vi "Init.vi"(5 "PathControl.lvclass":refnum<class "PathControl.lvclass">, 6 "Environmental classes":refnum<class "Instrument.lvclass">[](array[class]), 7 "XML Handler.lvclass":refnum<class "XML Handler.lvclass">, 8 "error in (no error)":errorcluster, 9 "Instruments to Use":T1(array[cluster]), 10 "Device.lvclass":refnum<class "Device.lvclass">, 11 "RF Powers in":refnum<class "RF Power.lvclass">) -> (0 "error out":errorcluster, 3 "RF Powers out":refnum<class "RF Power.lvclass">)   [LabVIEW 2020, in "RF Power.lvclass"]
doc: "Initializes the measurement.\nThis verifies that the instruments are present and adds them into the class data.\nIs also adds the xml handler into the class data."
uses:
  RF Power.lvclass
  Devices/Device.lvclass
  Instruments/Instrument.lvclass
  XML Handler/XML Handler.lvclass
  Path Control/PathControl.lvclass
  Harmonics/Controls/Init states.ctl
  Instruments/Signal Generator/Signal Generator.lvclass
  Instruments/Power Meter/Power Meter.lvclass
  Measurement.lvclass
  Harmonics/Harmonics.lvclass
panel:
  out "Current State":string
  out "Initializing Harmonic Measurement":u8(slide) scale=0.0..100.0
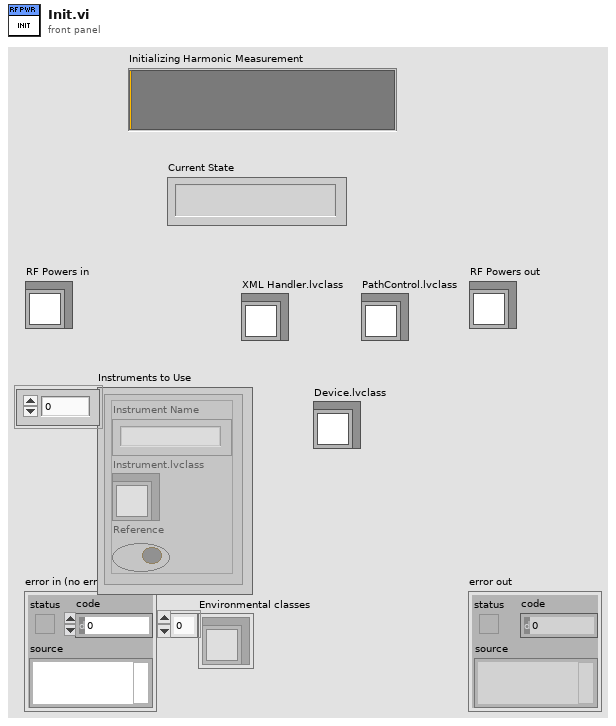
[diagram p1: front panel]
types:
  T1 = cluster{"Instrument Name":string, "Instrument.lvclass":refnum<class "Instrument.lvclass">, "Reference":bool}[]
  T2 = typedef "Harmonics.lvclass/Init states.ctl" = enum16{"Verify instruments", "Init Sweep Parameters", "Init Instruments", "Done"}
  T3 = typedef "RF Power.lvclass/Config info.ctl" = cluster{"Frequency (MHz)":string, "Power (dBm)":string, "Loop order":T4, "SG loss":bool, "PM loss":bool, "SG":i32}
  T4 = typedef "RF Power.lvclass/Loop order.ctl" = enum16{"Device -> Power -> Frequency", "Device -> Frequency -> Power"}
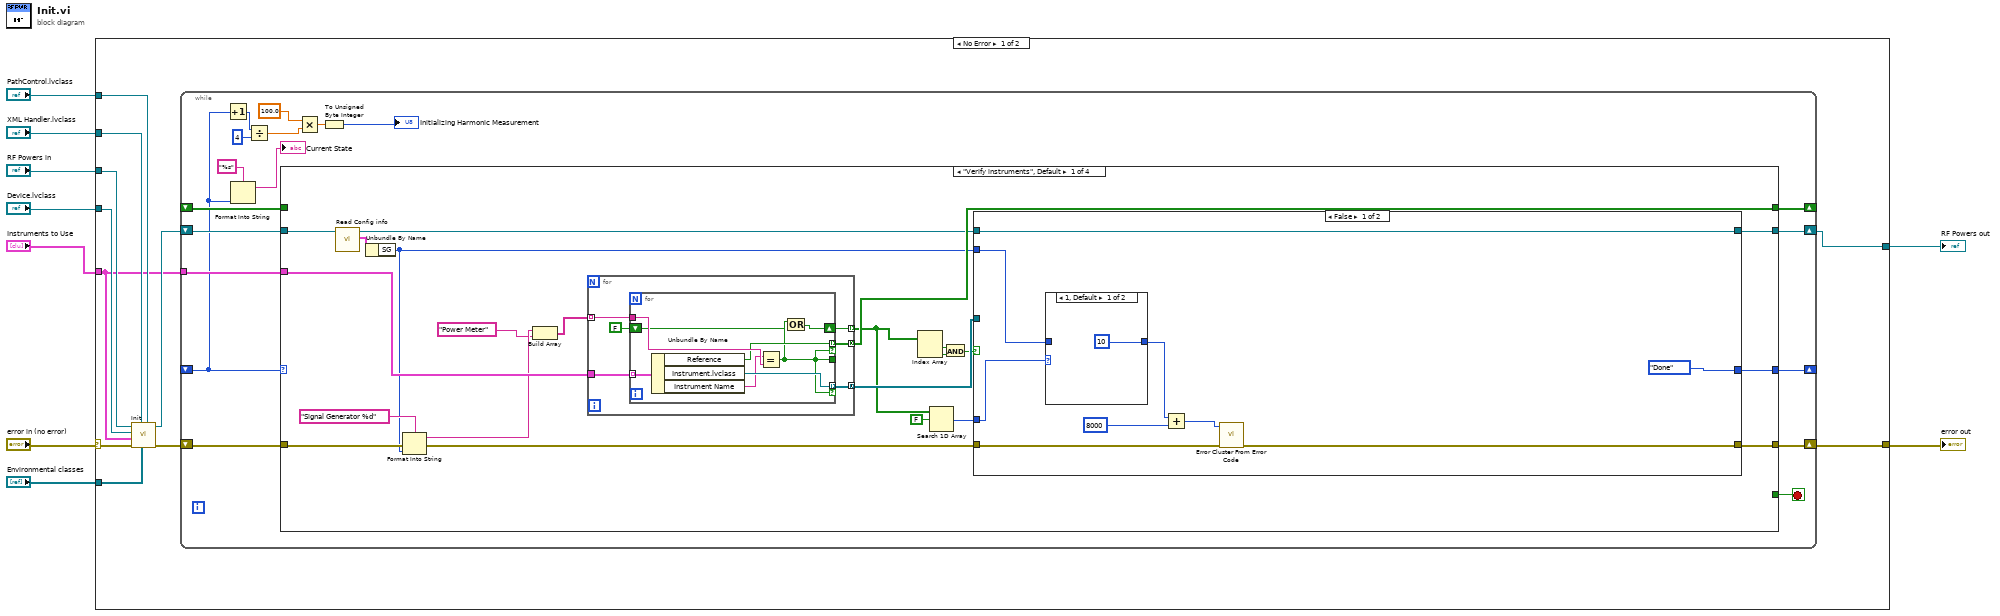
[diagram p0: block diagram]
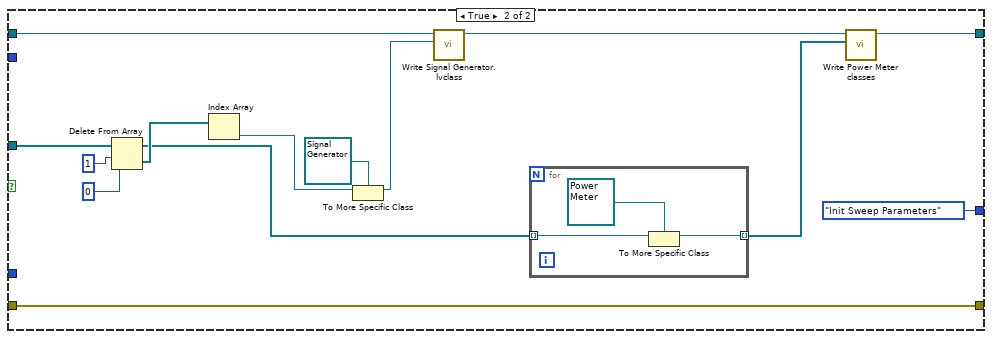
[diagram p3: hidden frame]
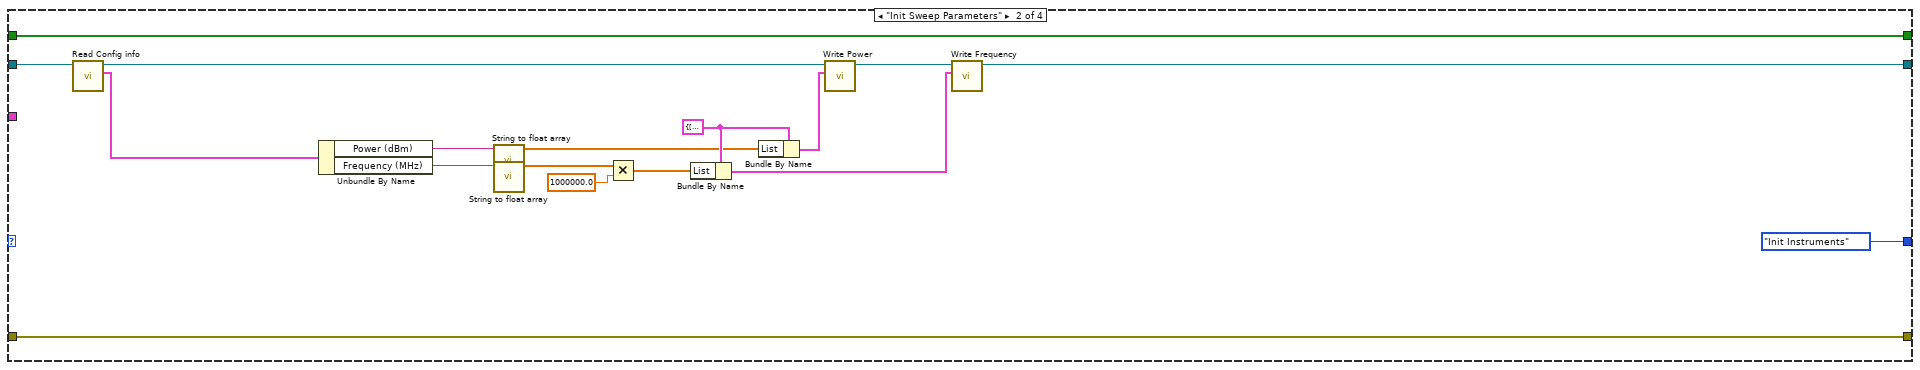
[diagram p4: hidden frame]
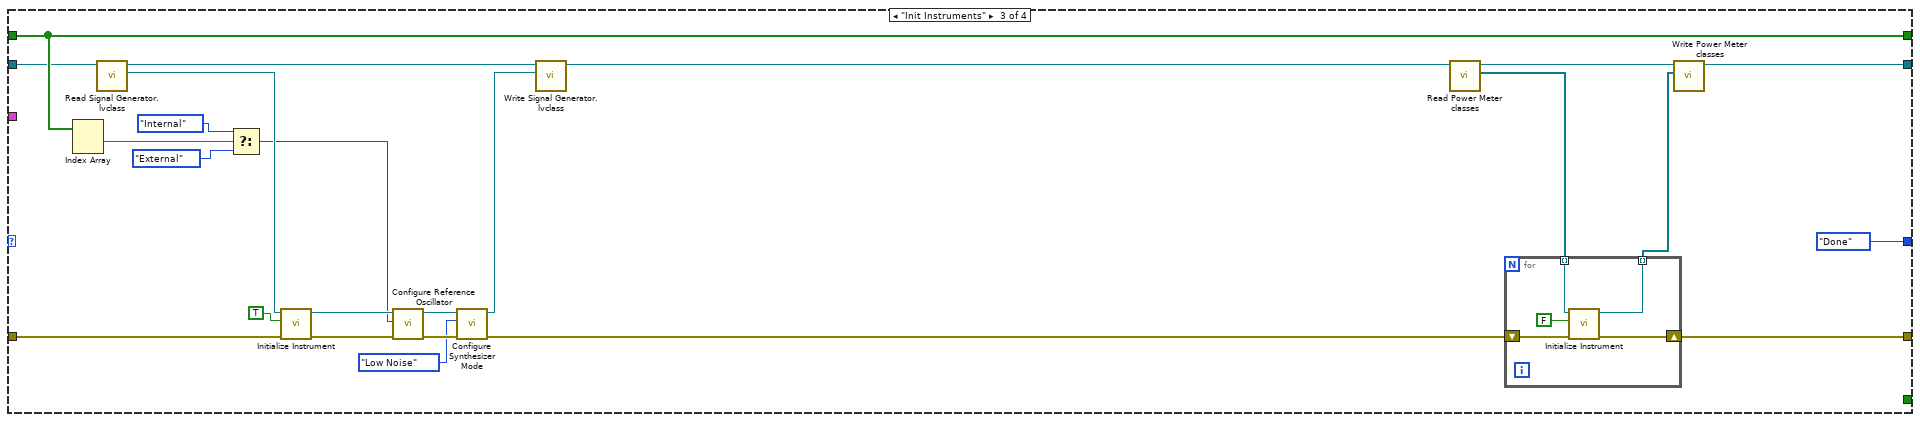
[diagram p5: hidden frame]
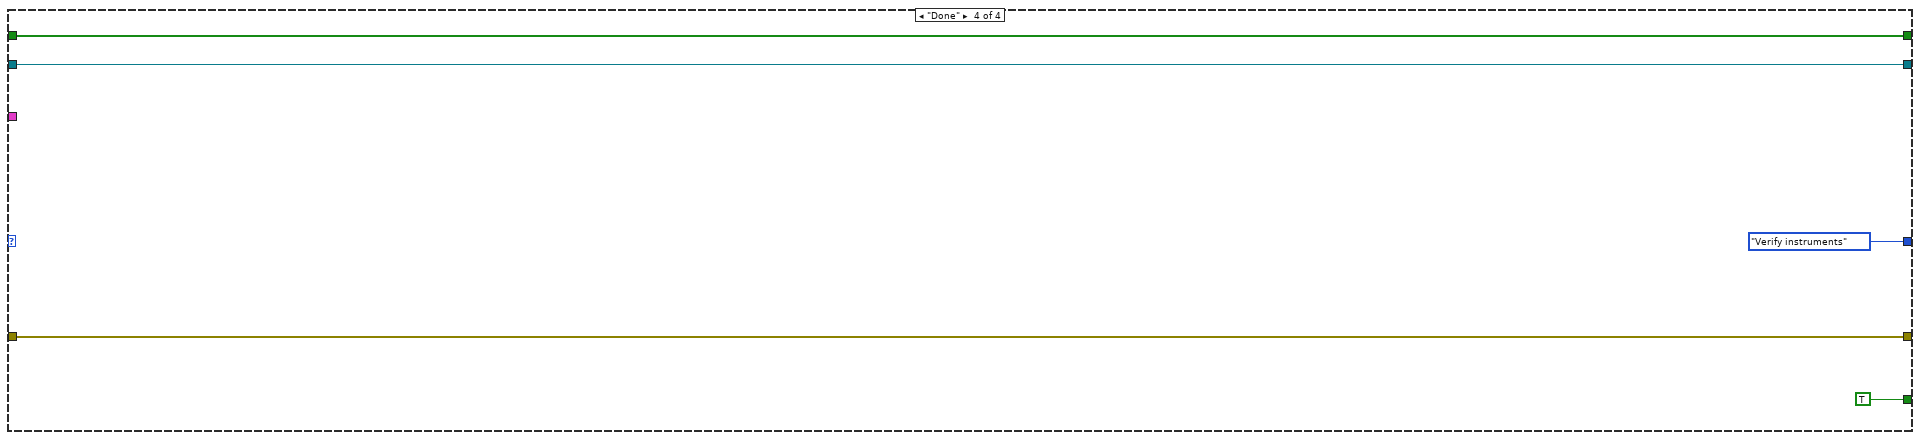
[diagram p6: hidden frame]
diagram:
  n1 = case shown="No Error" "error in (no error)" {
    selector: "error in (no error)" -> [w17 w154]
    tunnel: "PathControl.lvclass" -> [w20 _]
    tunnel: "Environmental classes" -> [w19 _]
    tunnel: "XML Handler.lvclass" -> [w18 _]
    tunnel: "Device.lvclass" -> [w16 _]
    tunnel: "RF Powers in" -> [w15 w155]
    tunnel: [w13 w154] -> w3
    tunnel: "Instruments to Use" -> [w11 _]
    tunnel: [w10 w155] -> w1
    frame No Error {
      n2 = call-parent "Init.vi"("PathControl.lvclass"=w20, "Environmental classes"=w19, "XML Handler.lvclass"=w18, "error in (no error)"=w17, "Instruments to Use"=w11, "Device.lvclass"=w16, "Measurements in"=w15) -> ("error out"=w14:errorcluster, "Measurements out"=w12:refnum<class "RF Power.lvclass">)  [unwired: 3 in]
      n3 = while {
        shift-right: [w34] -> w13
        shift-left: w14 -> [w35]
        tunnel: w11 -> [w38]
        shift-right: [w36] -> w10
        shift-left: w12 -> [w37]
        shift-right: [w32] -> _
        shift-left: _ -> [w27]
        shift-right: [w31] -> _
        shift-left: _ -> [w30]
        stop <- w33 stop-if-true
        n4 = Increment(x=w27) -> (x+1=w26:T2)
        n5 = Format Into String(format string="%s", w27) -> (resulting string=→"Current State":string)  [unwired: 2 in, 1 out]
        n6 = Divide(x=w26, y=4) -> (x/y=w24:dbl)
        n7 = case shown="\"Verify instruments\", Default" w27 {
          tunnel: w38 -> [w57 _ _ _]
          tunnel: w37 -> [w48 w104 w130 w149]
          tunnel: [w60 w106 w124 w149] -> w36
          tunnel: w35 -> [w44 w118 w142 w151]
          tunnel: [w59 w118 w131 w151] -> w34
          tunnel: [w58 Init_states."Init Instruments" Init_states."Done" Init_states."Verify instruments"] -> w32
          tunnel: [_ _ _ TRUE] -> w33
          tunnel: [w52 w116 w140 w153] -> w31
          tunnel: w30 -> [_ w116 w140 w153]
          frame "Verify instruments", Default {
            n8 = call-dynamic "Read Config info.vi"("RF Power in"=w48) -> ("Config info"=w45:T3, "RF Power out"=w47:refnum<class "RF Power.lvclass">)  [unwired: 9 in]
            n9 = Unbundle By Name(w45) -> ("SG"=w39:i32)
            n10 = Format Into String(format string="Signal Generator %d", error in=w44, w39) -> (resulting string=w42:string, error out=w43:errorcluster)  [unwired: 1 in]
            n11 = Build Array(w42, "Power Meter") -> (w40:string[])
            n12 = for {
              tunnel: [w66] -> w56 mode=concatenating
              tunnel: [w61] -> w51 mode=indexing
              tunnel: [w65] -> w52 mode=concatenating
              tunnel: w40 -> [w64] mode=indexing
              tunnel: w57 -> [w63]
              n13 = for {
                tunnel: w63 -> [w71] mode=indexing
                tunnel: w64 -> [w74]
                tunnel: [w73] -> w66 mode=indexing if=w68
                tunnel: [w68] -> _
                tunnel: [w72] -> w65 mode=indexing if=w68
                shift-right: [w69] -> w61
                shift-left: FALSE -> [w67]
                n14 = Unbundle By Name(w71) -> ("Reference"=w72:bool, "Instrument.lvclass"=w73:refnum<class "Instrument.lvclass">, "Instrument Name"=w70:string)
                n15 = Equal?(x=w70, y=w74) -> (x = y?=w68:bool)
                n16 = Or(x=w68, y=w67) -> (x .or. y?=w69:bool)
              }
            }
            n17 = Index Array(array=w51) -> (element #1=w55:bool, element #2=w54:bool)  [unwired: 2 in]
            n18 = Search 1D Array(1D array=w51, element=FALSE) -> (index of element=w49:i32)  [unwired: 1 in]
            n19 = And(x=w55, y=w54) -> (x .and. y?=w53:bool)
            n20 = case shown="False" w53 {
              tunnel: w56 -> [_ w93]
              tunnel: w47 -> [w83 w89]
              tunnel: [w83 w87] -> w60
              tunnel: w43 -> [w82 w96]
              tunnel: [w79 w96] -> w59
              tunnel: [Init_states."Done" Init_states."Init Sweep Parameters"] -> w58
              tunnel: w49 -> [w77 _]
              tunnel: w39 -> [w76 _]
              frame False {
                n21 = case shown="1, Default" w77 {
                  tunnel: w76 -> [_ w85]
                  tunnel: [10 ("y") w85] -> w75
                  frame 1, Default {
                  }
                  frame 0 {
                  }
                }
                n22 = Add(x=w75, y=8000) -> (x+y=w80:i32)
                n23 = call <vilib>:"Error Cluster From Error Code.vi"("error in (no error)"=w82, "error code (0)"=w80) -> ("error out"=w79:errorcluster)  [unwired: 7 in]
              }
              frame True {
                n24 = Delete From Array(array=w93, length=1, index=0) -> (deleted portion=w92:refnum<class "Instrument.lvclass">[], array with subset deleted=w91:refnum<class "Instrument.lvclass">[])
                n25 = Index Array(array=w92) -> (element=w99:refnum<class "Instrument.lvclass">)  [unwired: 1 in]
                n26 = To More Specific Class(target class=refnum<class "Signal Generator.lvclass"> refnum ("Signal Generator.lvclass"), reference=w99) -> (specific class reference=w90:refnum<class "Signal Generator.lvclass">)  [unwired: 1 in, 1 out]
                n27 = call-dynamic "Write Signal Generator.lvclass.vi"("Signal Generator.lvclass"=w90, "RF Power in"=w89) -> ("RF Power out"=w88:refnum<class "RF Power.lvclass">)  [unwired: 9 in]
                n28 = for {
                  tunnel: [w101] -> w86 mode=indexing
                  tunnel: w91 -> [w100] mode=indexing
                  n29 = To More Specific Class(target class=refnum<class "Power Meter.lvclass"> refnum ("Power Meter.lvclass"), reference=w100) -> (specific class reference=w101:refnum<class "Power Meter.lvclass">)  [unwired: 1 in, 1 out]
                }
                n30 = call-dynamic "Write Power Meter classes.vi"("Power Meter classes"=w86, "RF Power in"=w88) -> ("RF Power out"=w87:refnum<class "RF Power.lvclass">)  [unwired: 9 in]
              }
            }
          }
          frame "Init Sweep Parameters" {
            w117 = cluster{"List":dbl[], "Index":i32, "Last":bool} {"List"=[], "Index"=0, "Last"=FALSE} ("Power")
            n31 = call-dynamic "Read Config info.vi"("RF Power in"=w104) -> ("Config info"=w109:T3, "RF Power out"=w103:refnum<class "RF Power.lvclass">)  [unwired: 9 in]
            n32 = Unbundle By Name(w109) -> ("Power (dBm)"=w113:string, "Frequency (MHz)"=w111:string)
            n33 = call "String to float array.vi"("String"=w113) -> ("Array - Numeric"=w112:dbl[])  [unwired: 9 in, 1 out]
            n34 = call "String to float array.vi"("String"=w111) -> ("Array - Numeric"=w115:dbl[])  [unwired: 9 in, 1 out]
            n35 = Multiply(x=w115, y=1000000.0) -> (x*y=w110:dbl[])
            n36 = Bundle By Name(cluster=w117, "List"=w110) -> (w108:cluster{"List":dbl[], "Index":i32, "Last":bool})
            n37 = Bundle By Name(cluster=w117, "List"=w112) -> (w107:cluster{"List":dbl[], "Index":i32, "Last":bool})
            n38 = call-dynamic "Write Power.vi"("Power"=w107, "RF Power in"=w103) -> ("RF Power out"=w105:refnum<class "RF Power.lvclass">)  [unwired: 9 in]
            n39 = call-dynamic "Write Frequency.vi"("Frequency"=w108, "RF Power in"=w105) -> ("RF Power out"=w106:refnum<class "RF Power.lvclass">)  [unwired: 9 in]
          }
          frame "Init Instruments" {
            n40 = Index Array(array=w140) -> (element #1=w132:bool)  [unwired: 2 in, 1 out]
            n41 = call-dynamic "Read Signal Generator.lvclass.vi"("RF Power in"=w130) -> ("Signal Generator.lvclass"=w121:refnum<class "Signal Generator.lvclass">, "RF Power out"=w122:refnum<class "RF Power.lvclass">)  [unwired: 9 in]
            n42 = Select(t=enum16{"Internal", "External"}."Internal" ("Reference Mode"), s=w132, f=enum16{"Internal", "External"}."External") -> (s? t:f=w120:enum16{"Internal", "External"})
            n43 = call-dynamic "Initialize Instrument.vi"("error in (no error)"=w142, "Reset"=TRUE, "Instrument in"=w121) -> ("error out"=w137:errorcluster, "Instrument out"=w139:refnum<class "Signal Generator.lvclass">)  [unwired: 7 in]
            n44 = call-dynamic "Configure Reference Oscillator.vi"("error in (no error)"=w137, "Reference Mode"=w120, "Signal Generator in"=w139) -> ("error out"=w138:errorcluster, "Signal Generator out"=w136:refnum<class "Signal Generator.lvclass">)  [unwired: 7 in]
            n45 = call-dynamic "Configure Synthesizer Mode.vi"("error in (no error)"=w138, "Synthesizer Mode"=enum16{"Normal", "Low Noise"}."Low Noise", "Signal Generator in"=w136) -> ("error out"=w123:errorcluster, "Signal Generator out"=w129:refnum<class "Signal Generator.lvclass">)  [unwired: 7 in]
            n46 = call-dynamic "Write Signal Generator.lvclass.vi"("Signal Generator.lvclass"=w129, "RF Power in"=w122) -> ("RF Power out"=w127:refnum<class "RF Power.lvclass">)  [unwired: 9 in]
            n47 = call-dynamic "Read Power Meter classes.vi"("RF Power in"=w127) -> ("Power Meter classes"=w128:refnum<class "Power Meter.lvclass">[], "RF Power out"=w126:refnum<class "RF Power.lvclass">)  [unwired: 9 in]
            n48 = for {
              tunnel: w128 -> [w147] mode=indexing
              tunnel: [w144] -> w125 mode=indexing
              shift-right: [w145] -> w131
              shift-left: w123 -> [w148]
              n49 = call-dynamic "Initialize Instrument.vi"("error in (no error)"=w148, "Reset"=FALSE, "Instrument in"=w147) -> ("error out"=w145:errorcluster, "Instrument out"=w144:refnum<class "Power Meter.lvclass">)  [unwired: 7 in]
            }
            n50 = call-dynamic "Write Power Meter classes.vi"("Power Meter classes"=w125, "RF Power in"=w126) -> ("RF Power out"=w124:refnum<class "RF Power.lvclass">)  [unwired: 9 in]
          }
          frame "Done" {
          }
        }
        n51 = Multiply(x=100.0 ("y"), y=w24) -> (x*y=w22:dbl)
        n52 = To Unsigned Byte Integer(number=w22) -> (unsigned 8bit integer=→"Initializing Harmonic Measurement":u8)
      }
    }
    frame Error {
    }
  }
  "error out" <- w3
  "RF Powers out" <- w1
